vi "Change Date.vi"(8 "error in (no error)":errorcluster, 10 "Date":timestamp, 11 "VISA resource name":refnum<visa-resource-name>) -> (0 "error out":errorcluster, 3 "VISA resource name out":refnum<visa-resource-name>)   [LabVIEW 2017, in "Sefram DAS220.lvlib"]
doc: "Change the date of the device."
uses:
  <instrlib>/Sefram DAS220/Sefram DAS220.lvlib
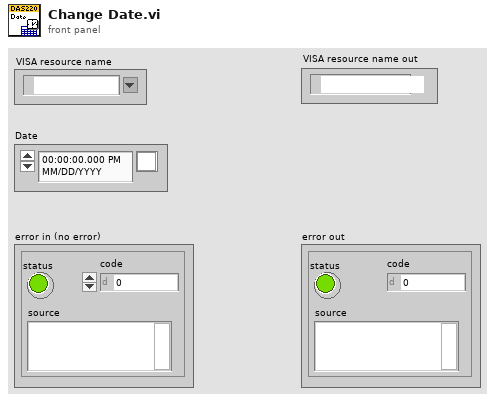
[diagram p1: front panel]
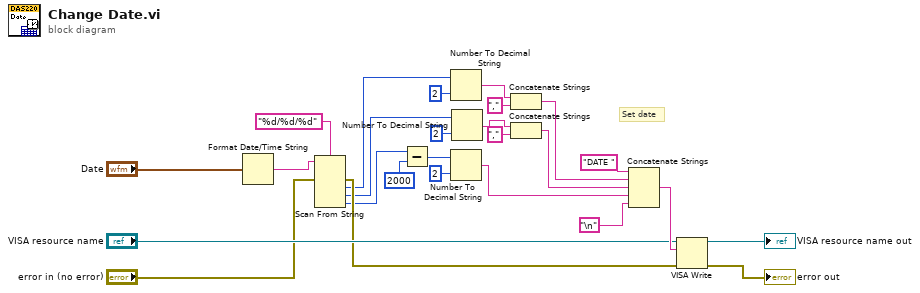
[diagram p0: block diagram]
diagram:
  # "Set date"
  n1 = Format Date/Time String(seconds (now)="Date") -> (date/time string=w5:string)  [unwired: 2 in]
  n2 = Scan From String(format string="%d/%d/%d", input string=w5, error in="error in (no error)") -> (error out=w6:errorcluster, output 1=w4:i32, output 2=w3:i32, output 3=w2:i32)  [unwired: 4 in, 2 out]
  n3 = Subtract(x=w2, y=2000) -> (x-y=w9:i32)
  n4 = Number To Decimal String(number=w4, width (-)=i16 2) -> (decimal integer string=w17:string)
  n5 = Number To Decimal String(number=w9, width (-)=i16 2) -> (decimal integer string=w11:string)
  n6 = Number To Decimal String(number=w3, width (-)=i16 2) -> (decimal integer string=w13:string)
  n7 = Concatenate Strings(w17, "," ("string")) -> (w15:string)
  n8 = Concatenate Strings(w13, "," ("string")) -> (w12:string)
  n9 = Concatenate Strings("DATE " ("string"), w15, w12, w11, "\n") -> (w26:string)
  n10 = VISA Write(VISA resource name="VISA resource name", write buffer=w26, error in (no error)=w6) -> (VISA resource name out=→"VISA resource name out":refnum<visa-resource-name>, error out=→"error out":errorcluster)  [unwired: 1 out]
